vi "CSC_GetVecInGCS.vi"(8 "error in (no error)":errorcluster, 9 "Body ID":i32, 10 "xyz":dbl[](array[numeric])=[0.0, 0.0, 0.0], 11 "CSC":refnum<class "CableSerialChain.lvclass">) -> (0 "error out":errorcluster, 2 "PointInGCS":dbl[](array[numeric]), 3 "CSC":refnum<class "CableSerialChain.lvclass">)   [LabVIEW 2015, in "CableSerialChain.lvclass"]
uses:
  CableSerialChain.lvclass
  CableSerialChain.lvclass/CableSerialChain.ctl
  <vilib>/Analysis/BLAS.llb/gemv - General Matrix-Vector Product.vi
  <vilib>/Analysis/BLAS.llb/dgemv - General Matrix-Vector Product (DBL).vi
  <vilib>/Utility/error.llb/Error Cluster From Error Code.vi
  Body/Bodies.lvclass
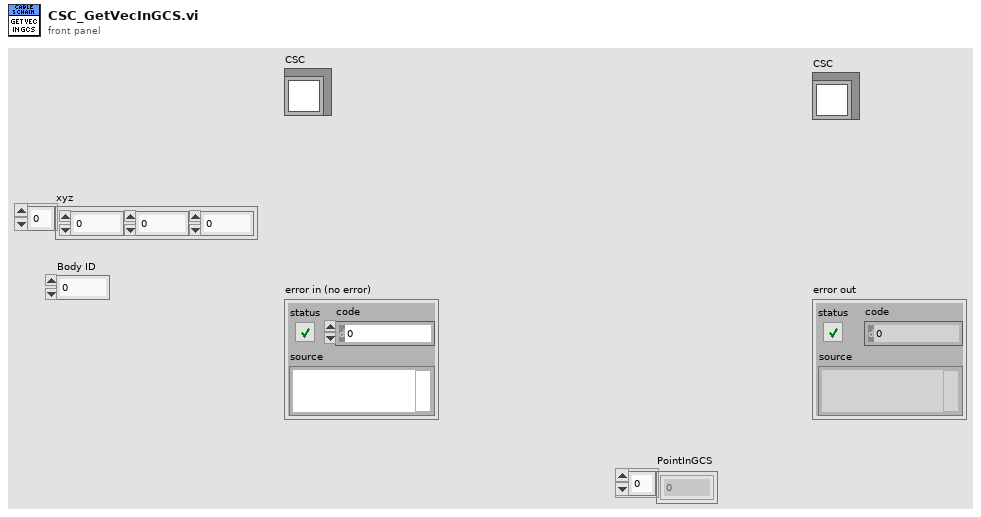
[diagram p1: front panel]
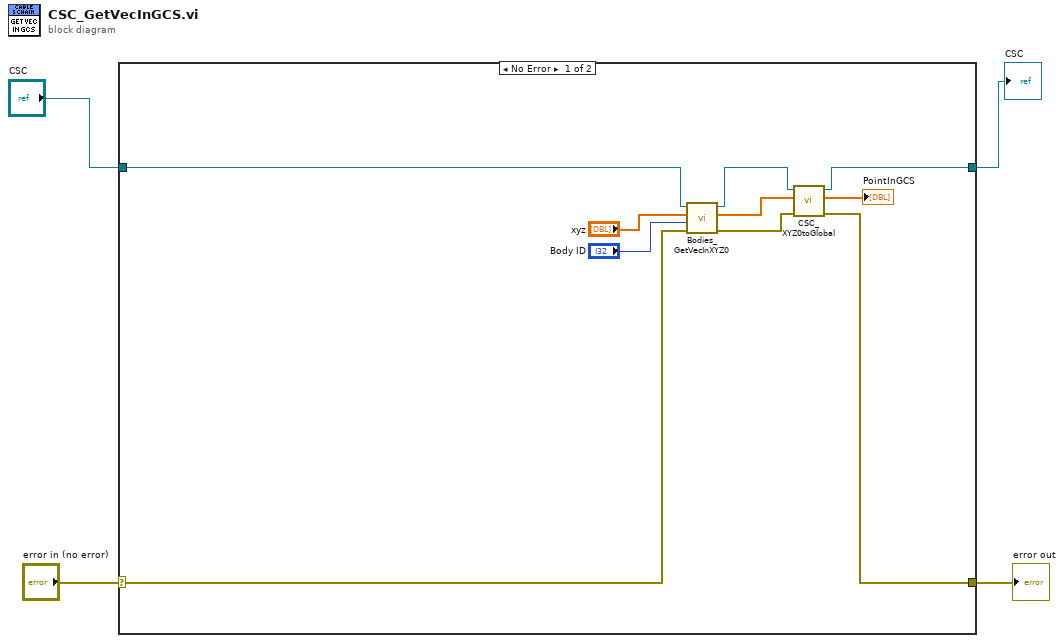
[diagram p0: block diagram]
diagram:
  n1 = case shown="No Error" "error in (no error)" {
    selector: "error in (no error)" -> [w14 w16]
    tunnel: "CSC" -> [w7 w15]
    tunnel: [w8 w16] -> w3
    tunnel: [w5 w15] -> w1
    frame No Error {
      n2 = call "Bodies_GetVecInXYZ0.vi"("error in (no error)"=w14, "Body ID"="Body ID", "Vector"="xyz", "Bodies.lvclass"=w7) -> ("error out"=w9:errorcluster, "Vector in GCS"=w11:dbl[], "Bodies.lvclass 2"=w6:refnum<class "CableSerialChain.lvclass">)  [unwired: 5 in]
      n3 = call "CSC_XYZ0toGlobal.vi"("error in (no error)"=w9, "Pin"=w11, "CSC In"=w6) -> ("error out"=w8:errorcluster, "Pout"=→"PointInGCS":dbl[], "CSC Oout"=w5:refnum<class "CableSerialChain.lvclass">)  [unwired: 5 in, 1 out]
    }
    frame Error {
    }
  }
  "error out" <- w3
  "CSC" <- w1
